vi "test_section_dP.vi"(0 "dP Voltage":dynamicdata(graph), 1 "Offset[Pa]":dbl) -> (2 "dP":dbl, 3 "Adj dP":dbl, 4 "Adj dP Array":dynamicdata(graph))   [LabVIEW 2017]
uses:
  <vilib>/express/express arith-compare/Formula/XNode/ExpressFormulaBlockNode.xnode
  <vilib>/express/express shared/transition.llb/Dynamic To Waveform Array.vi
  <vilib>/express/express arith-compare/Formula/Block/exnFormulaBlock how many pts in the wave.vi
  <vilib>/express/express shared/ex_Modify Signal Name.vi
  <vilib>/express/express shared/transition.llb/Waveform Array To Dynamic.vi
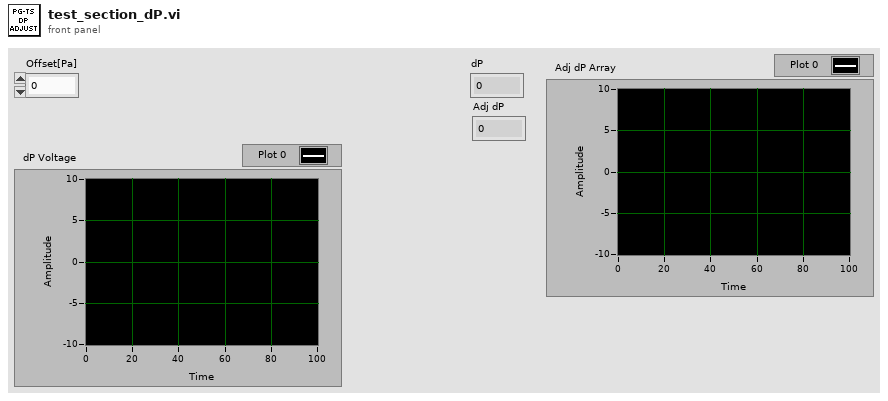
[diagram p1: front panel]
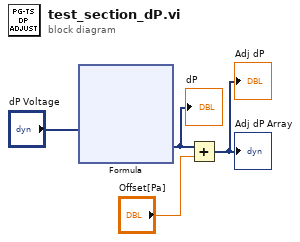
[diagram p0: block diagram]
diagram:
  n1 = xnode "Formula"("V"="dP Voltage") -> ("Result"=w4:dynamicdata)  [unwired: 1 in, 1 out]
  "dP" <- w4
  n2 = Add(x=w4, y="Offset[Pa]") -> (x+y=→"Adj dP" →"Adj dP Array":dynamicdata)
